vi "SetVoltage.vi"(3 "Voltage":dbl, 4 "error in":errorcluster, 5 "connection ID":refnum<k5>) -> (0 "False":bool, 1 "error out":errorcluster, 2 "connection ID out":refnum<k5>)   [LabVIEW 2013]
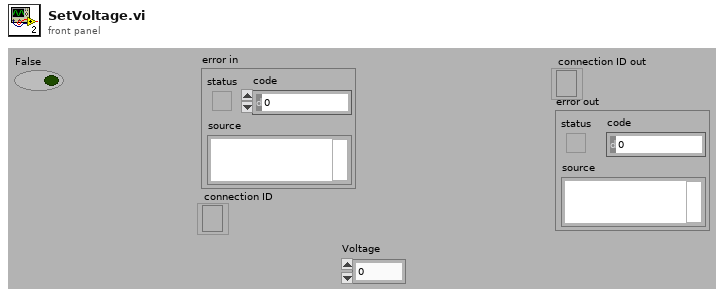
[diagram p1: front panel]
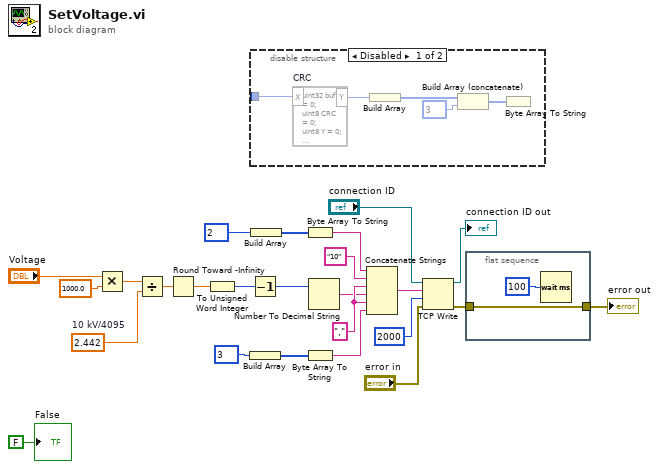
[diagram p0: block diagram]
diagram:
  w14 = 2.442  # 10 kV/4095
  w16 = "," ("string")
  n1 = Multiply(x="Voltage", y=1000.0) -> (x*y=w9:dbl)
  n2 = Divide(x=w9, y=w14) -> (x/y=w7:dbl)
  n3 = Round Toward -Infinity(1:w7) -> (0:w6:dbl)
  n4 = To Unsigned Word Integer(number=w6) -> (unsigned 16bit integer=w13:u16)
  n5 = Decrement(x=w13) -> (x-1=w8:u16)
  n6 = Build Array(u8 3 ("y")) -> (w1:u8[])
  n7 = disable-structure shown="Disabled" {
    disable-tunnel: _ -> [w26 _]
    frame Disabled {
      n8 = formula code="uInt32 buf = 0;\nuInt8 CRC = 0;\nuInt8 Y = 0;\n\nbuf = 0x31 + 0x30  + X + 0x2C;\nbuf = ~ buf;\nbuf = buf & 0x000000FF;\nCRC = buf;\nCRC &= 0x7F;\nCRC |= 0x40;\nCRC++;\nY = CRC;" "CRC"("X"=w26) -> ("Y"=w28:u8)
      n9 = Build Array(w28) -> (w27:u8[])
      n10 = Build Array (concatenate)(w27, u8 3 ("y")) -> (w29:u8[])
      n11 = Byte Array To String(unsigned byte array=w29) -> ()  [unwired: 1 out]
    }
    frame Enabled {
    }
  }
  n12 = Build Array(u8 2 ("y")) -> (w19:u8[])
  n13 = Byte Array To String(unsigned byte array=w19) -> (string=w18:string)
  n14 = Byte Array To String(unsigned byte array=w1) -> (string=w2:string)
  n15 = Number To Decimal String(number=w8) -> (decimal integer string=w12:string)  [unwired: 1 in]
  n16 = Concatenate Strings(w18, "10" ("string"), w16, w12, w16, w2) -> (w15:string)
  n17 = TCP Write(connection ID="connection ID", data in=w15, error in (no error)="error in", 9:2000 ("timeout ms (25000)")) -> (connection ID out=→"connection ID out":refnum<k5>, error out=w4:errorcluster)  [unwired: 1 out]
  n18 = flat-sequence {
    tunnel: [w32] -> w5
    tunnel: w4 -> [w32]
    frame #0 {
      n19 = Wait (ms)(milliseconds to wait=u32 100) -> ()  [unwired: 1 out]
    }
  }
  "error out" <- w5
  "False" <- FALSE
